vi "Packed Library Path.vi"(3 "error in (no error)":errorcluster, 5 "vi reference":refnum<vi>) -> (0 "error out":errorcluster, 1 "packed library path":path, 2 "vi reference out":refnum<vi>)   [LabVIEW 2026, in "NI_PackedLibraryUtility.lvlib"]
doc: "Returns the path to a <a href=\"nihelplauncher://docs/csh?context=lvcore_lvconcepts_packed_libraries\">packed project library</a> for the VI you specify in <strong>vi reference</strong>."
uses:
  NI_PackedLibraryUtility.lvlib
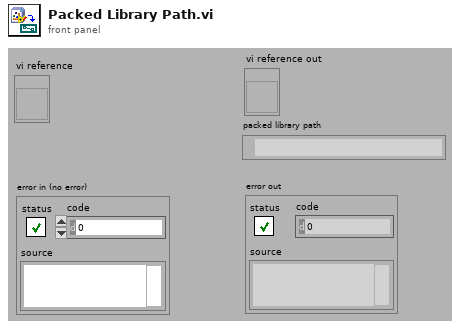
[diagram p1: front panel]
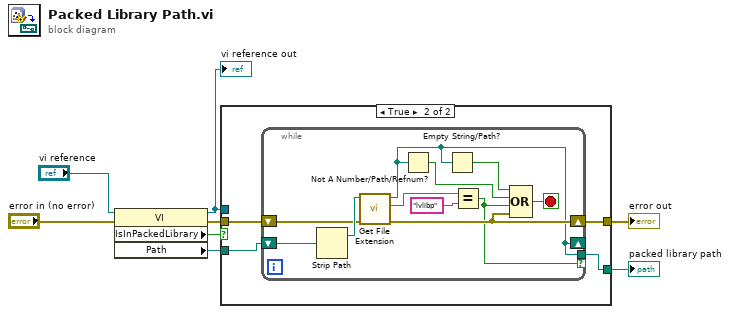
[diagram p0: block diagram]
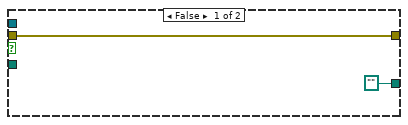
[diagram p2: hidden frame]
diagram:
  n1 = property class="VI"(reference="vi reference", error in="error in (no error)") -> (reference out=w1:refnum<vi>, error out=w7:errorcluster, "IsInPackedLibrary"=w8:bool, "Path"=w2:path)
  "vi reference out" <- w1
  n2 = case shown="True" w8 {
    tunnel: w7 -> [w9 w13]
    tunnel: [path "" w11] -> w6
    tunnel: [w9 w12] -> w4
    tunnel: w1 -> [_ _]
    tunnel: w2 -> [_ w14]
    frame False {
    }
    frame True {
      n3 = while {
        shift-right: [w16] -> _
        shift-left: w14 -> [w25]
        shift-right: [w17] -> w12
        shift-left: w13 -> [w21]
        tunnel: [w16] -> w11 if=w15
        stop <- w20 stop-if-true
        n4 = Strip Path(path=w25) -> (stripped path=w24:path)  [unwired: 1 out]
        n5 = call "Get File Extension.vi"("error in (no error)"=w21, "file"=w24) -> ("error out"=w17:errorcluster, "lowercase file extension"=w23:string, "dup file"=w16:path)  [unwired: 5 in, 2 out]
        n6 = Not A Number/Path/Refnum?(number/path/refnum=w16) -> (NaN/Path/Refnum?=w19:bool)
        n7 = Empty String/Path?(string/path=w16) -> (empty?=w18:bool)
        n8 = Equal?(x=w23, y="lvlibp") -> (x = y?=w15:bool)
        n9 = Compound Arithmetic op=OR(w18, w19, w15, w17) -> (w20:bool)
      }
    }
  }
  "packed library path" <- w6
  "error out" <- w4
